vi "ConvertGoop3ToGoop4_UpdateGetAttributes.vi"(8 "error in (no error)":errorcluster, 10 "BaseClasses":path[](array[path]), 11 "ViRef":refnum<vi>) -> (0 "error out":errorcluster, 3 "ViRefOut":refnum<vi>)   [LabVIEW 2014]
uses:
  <resource>/Framework/Providers/Open_GDS/ClassProviders/Common/ScriptingFunctions/Scripting_FollowWireDownStreams_StopCriteria.ctl
panel:
  out "BundlerNames":cluster{"FullElemNms[]":cluster{string[]}[]}[](array[cluster])
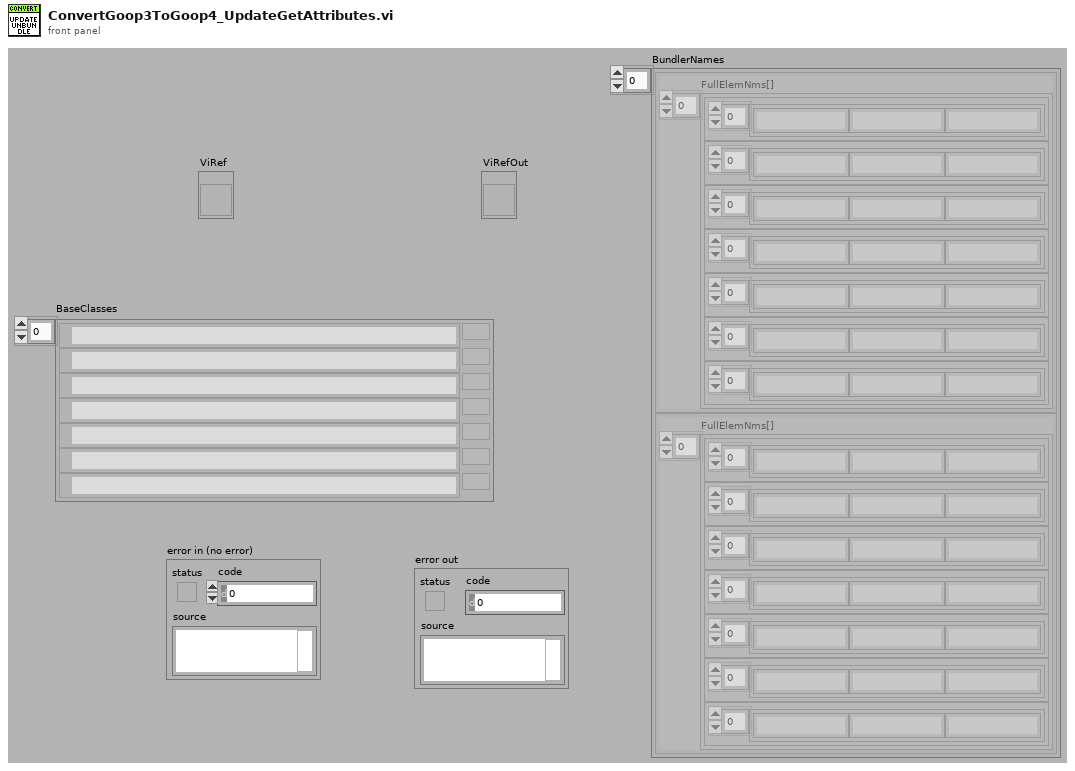
[diagram p1: front panel]
types:
  T1 = typedef "Scripting_FollowWireDownStreams_StopCriteria.ctl" = cluster{"ReachedANyOfTheseNodes":refnum<vi>[], "NodeType":string[], "VINames":string[], "AddTheseNodes":bool, "ALsoSerachOtherDrainNodes":bool}
  T2 = cluster{"Bundlers":refnum<vi>, "BundlersSourceTerms":refnum<vi>[], "BundlersClassBelongingsOut":i32[], "Bundler":refnum<vi>}[]
  T3 = cluster{"WhileLoop":refnum<vi>, refnum<vi>[], i32[], "WhileLoop":refnum<vi>}
  T4 = cluster{"WhileLoop":refnum<vi>, "BundlersSourceTerms":refnum<vi>[], "BundlersClassBelongingsOut":i32[], "WhileLoop":refnum<vi>}[]
  T5 = cluster{"WhileLoop":refnum<vi>, "BundlersSourceTerms":refnum<vi>[], "BundlersClassBelongingsOut":i32[], "WhileLoop":refnum<vi>}
  T6 = cluster{"Bundlers":refnum<vi>, "BundlersSourceTerms":refnum<vi>[], "BundlersClassBelongingsOut":i32[], "Bundler":refnum<vi>}
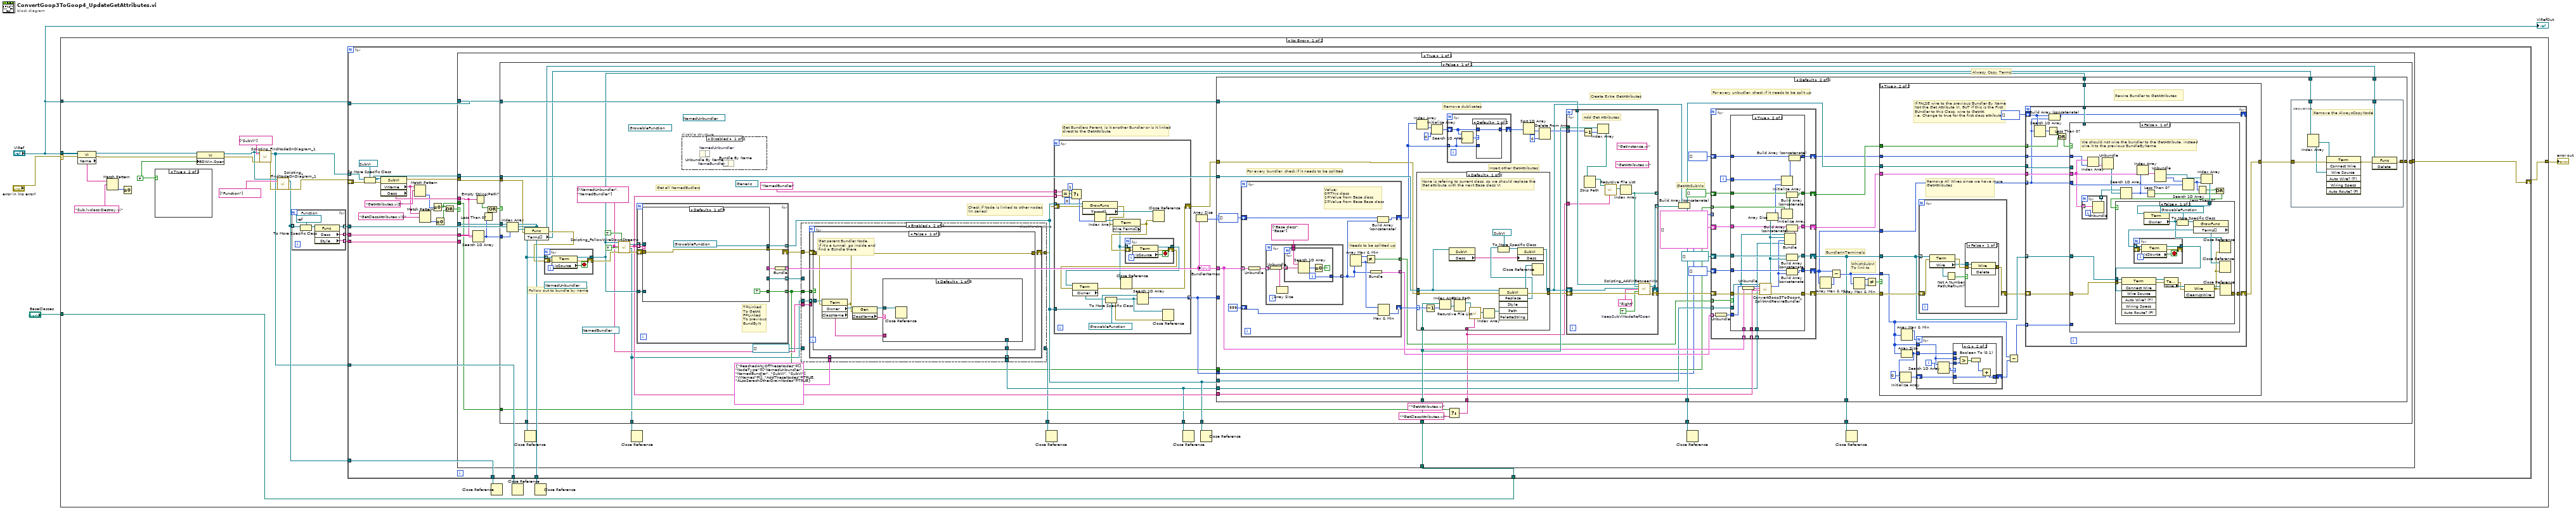
[diagram p0: block diagram]
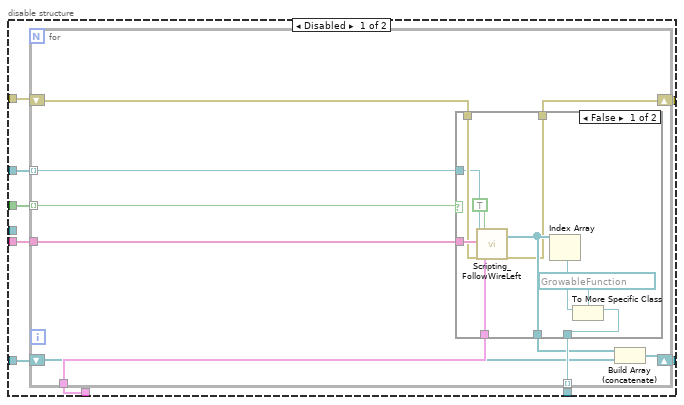
[diagram p4: hidden frame]
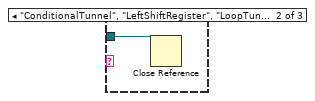
[diagram p6: hidden frame]
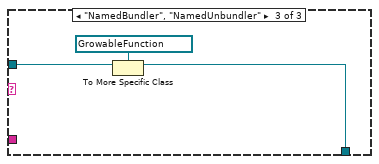
[diagram p7: hidden frame]
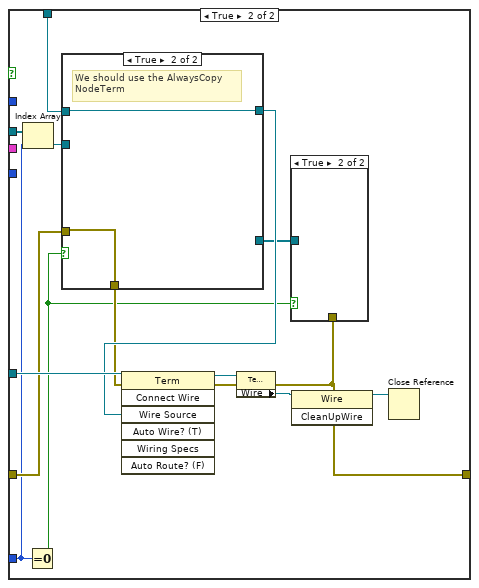
[diagram p13: hidden frame]
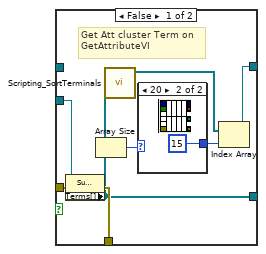
[diagram p14: hidden frame]
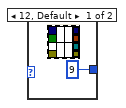
[diagram p15: hidden frame]
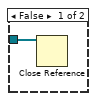
[diagram p16: hidden frame]
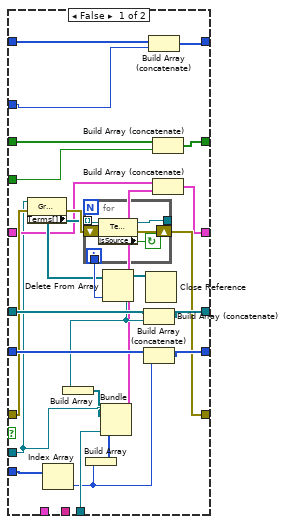
[diagram p18: hidden frame]
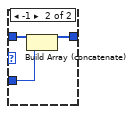
[diagram p19: hidden frame]
diagram:
  n1 = case shown="No Error" "error in (no error)" {
    selector: "error in (no error)" -> [w6 w587]
    tunnel: [w28 w587] -> w4
    tunnel: "ViRef" -> [w9 _]
    tunnel: "BaseClasses" -> [w15 _]
    tunnel: "ViRef" -> [w14 _]
    frame No Error {
      w5 = FALSE
      n2 = property class="VI"(reference=w9, error in=w6) -> (reference out=w8:refnum<vi>, error out=w7:errorcluster, "Name"=w12:string)
      n3 = Match Pattern(string=w12, regular expression="Sub.lvclass:Destroy.vi") -> (offset past match=w10:i32)  [unwired: 1 in, 3 out]
      n4 = Greater Or Equal To 0?(x=w10) -> ()  [unwired: 1 out]
      n5 = case shown="True" w5 {
        frame False {
        }
        frame True {
        }
      }
      n6 = property class="VI"(reference=w8, error in=w7, "BDWin.Open"=w5) -> (reference out=w26:refnum<vi>, error out=w27:errorcluster)
      n7 = call <resource>:"Scripting_FindNodeOnDiagram_1.vi"("ViRef(Ignored If Not Wired)"=w26, "NodeTypesToSearchFor"=string[] ["SubVI"], "error in (no error)"=w27) -> ("Nodes"=w13:refnum<vi>[], "error out"=w24:errorcluster)  [unwired: 15 in]
      n8 = call <resource>:"Scripting_FindNodeOnDiagram_1.vi"("ViRef(Ignored If Not Wired)"=w26, "NodeTypesToSearchFor"=string[] ["Function"], "error in (no error)"=w24) -> ("Nodes"=w19:refnum<vi>[], "error out"=w23:errorcluster)  [unwired: 15 in]
      n9 = for {
        tunnel: w19 -> [w33] mode=indexing
        tunnel: [w32] -> w22 mode=indexing
        tunnel: [w31] -> w21 mode=indexing
        tunnel: [w30] -> w16 mode=indexing
        w34 = refnum<vi> refnum  # Function
        n10 = To More Specific Class(target class=w34, reference=w33) -> (specific class reference=w35:refnum<vi>)  [unwired: 1 in, 1 out]
        n11 = property class="Func"(reference=w35) -> (reference out=w31:refnum<vi>, "Desc"=w32:string, "Style"=w30:string)  [unwired: 1 in, 1 out]
      }
      n12 = for {
        tunnel: w13 -> [w59] mode=indexing
        shift-right: [w46] -> w28
        shift-left: w23 -> [w57]
        tunnel: w22 -> [w50]
        tunnel: w21 -> [w49]
        tunnel: [w49] -> w20
        tunnel: w19 -> [w48]
        tunnel: [w48] -> w18
        tunnel: w13 -> [w47]
        tunnel: [w47] -> w17
        tunnel: w16 -> [w45]
        tunnel: w15 -> [w44]
        tunnel: w14 -> [w43]
        n13 = To More Specific Class(target class=refnum<vi> refnum ("WhileLoop"), reference=w59, error in=w57) -> (specific class reference=w56:refnum<vi>, error out=w55:errorcluster)
        n14 = property class="SubVI"(reference=w56, error in=w55) -> (reference out=w53:refnum<vi>, error out=w52:errorcluster, "VIName"=w36:string, "Desc"=w51:string)
        n15 = Match Pattern(string=w36, regular expression="GetAttributes.vi$") -> (offset past match=w39:i32)  [unwired: 1 in, 3 out]
        n16 = Match Pattern(string=w36, regular expression="GetClassAttributes.vi$") -> (offset past match=w41:i32)  [unwired: 1 in, 3 out]
        n17 = Greater Or Equal To 0?(x=w39) -> (x >= 0?=w37:bool)
        n18 = Greater Or Equal To 0?(x=w41) -> (x >= 0?=w40:bool)
        n19 = Or(x=w37, y=w40) -> (x .or. y?=w38:bool)
        n20 = case shown="True" w38 {
          tunnel: w53 -> [w79 _]
          tunnel: w52 -> [w78 w586]
          tunnel: [w77 w586] -> w46
          tunnel: w51 -> [w72 _]
          tunnel: w50 -> [w76 _]
          tunnel: w49 -> [w75 _]
          tunnel: w45 -> [_ _]
          tunnel: w44 -> [w74 _]
          tunnel: w43 -> [w73 _]
          tunnel: w37 -> [w63 _]
          frame True {
            n21 = Search 1D Array(1D array=w76, element=w72) -> (index of element=w70:i32)  [unwired: 1 in]
            n22 = Empty String/Path?(string/path=w72) -> (empty?=w71:bool)
            n23 = Less Than 0?(x=w70) -> (x < 0?=w69:bool)
            n24 = Compound Arithmetic op=OR(w71, w69) -> (w68:bool)
            n25 = case shown="False" w68 {
              tunnel: w79 -> [w114 _]
              tunnel: w78 -> [w96 w585]
              tunnel: [w109 w585] -> w77
              tunnel: w75 -> [w119 _]
              tunnel: w74 -> [w112 _]
              tunnel: w73 -> [w113 _]
              tunnel: w70 -> [w110 _]
              tunnel: [w107 _] -> w67
              tunnel: [w97 _] -> w66
              tunnel: [w106 _] -> w65
              tunnel: [w105 _] -> w64
              tunnel: w63 -> [w94 _]
              tunnel: [w90 _] -> w62
              tunnel: [w85 _] -> w61
              tunnel: [w84 _] -> w60
              frame False {
                (unwired) refnum<vi> refnum ("Owner")
                (unwired) refnum<vi> refnum ("WhileLoop")
                (unwired) refnum<vi> refnum ("WhileLoop")
                (unwired) refnum<vi> refnum ("WhileLoop")
                w88 = string[] ["NamedUnbundler", "NamedBundler"]
                (unwired) refnum<vi> refnum ("WhileLoop")
                # "Check if Node is linked to other nodes\n(In series)"
                # "Get Bundlers Parent, is it another Bundler or is it linked\ndirect to the GetAttribute"
                # "Alwasy Copy Terms"
                # "Get all NamedBudlers"
                # "Follow out to bundle by name"
                n26 = Index Array(array=w119, index=w110) -> (element=w118:refnum<vi>)
                n27 = property class="Func"(reference=w118, error in=w96) -> (reference out=w108:refnum<vi>, error out=w116:errorcluster, "Terms[]"=w107:refnum<vi>[])
                n28 = for {
                  tunnel: w107 -> [w533] mode=indexing
                  tunnel: [w532] -> w102
                  shift-right: [w529] -> w115
                  shift-left: w116 -> [w530]
                  stop <- w531 stop-if-true
                  n29 = property class="Term"(reference=w533, error in=w530) -> (reference out=w532:refnum<vi>, error out=w529:errorcluster, "IsSource"=w531:bool)
                }
                n30 = call <resource>:"Scripting_FollowWireDownStreams.vi"("Term Refnum"=w102, "NodeTypesToFind"=w88, "CreateParentTerminals(False)"=TRUE, "error in"=w115, "MainitainDataType"=TRUE ("MainitainDateType(True)")) -> ("Nodes"=w111:refnum<vi>[], "NodeTypes"=w101:string[], "ParentTerminal"=w84:refnum<vi>[], "error out"=w117:errorcluster)  [unwired: 11 in]
                n31 = for {
                  tunnel: w111 -> [w543] mode=indexing
                  shift-right: [w541] -> w89
                  shift-left: w117 -> [w542]
                  tunnel: [w539] -> w104 mode=indexing
                  tunnel: [w537] -> w97 mode=indexing
                  tunnel: w101 -> [w538] mode=indexing
                  tunnel: w102 -> [w536]
                  tunnel: [w535] -> w83 mode=indexing
                  tunnel: [w534] -> w82 mode=indexing
                  # "T=Linked\nTo GetAt\nF=Linked\nTo previous\nBundByN"
                  n32 = case shown="Default" w538 {
                    tunnel: w543 -> [_ w565 w584]
                    tunnel: w542 -> [w546 w561 w581]
                    tunnel: [w546 w560 w580] -> w541
                    tunnel: [_ w559 w579] -> w540
                    tunnel: [refnum<vi> refnum ("WhileLoop") w556 w576] -> w537
                    tunnel: w536 -> [_ w554 w574]
                    tunnel: [TRUE w552 w572] -> w535
                    tunnel: [_ w547 w568] -> w534
                    frame Default {
                    }
                    frame "NamedUnbundler" {
                      (unwired) refnum<vi> refnum ("WhileLoop")
                      n33 = To More Specific Class(target class=refnum<vi> refnum ("WhileLoop"), reference=w565, error in=w561) -> (specific class reference=w563:refnum<vi>, error out=w562:errorcluster)
                      n34 = property class="NmdUnbndl"(reference=w563, error in=w562) -> (reference out=w558:refnum<vi>, error out=w560:errorcluster, "FullElemNms[]"=w559:cluster{string[]}[], "Terms[]"=w551:refnum<vi>[])
                      n35 = Delete From Array(array=w551, index=0) -> (deleted portion=w548:refnum<vi>, array with subset deleted=w550:refnum<vi>[])  [unwired: 1 in]
                      n36 = property class="Term"(reference=w548) -> (reference out=w547:refnum<vi>, "Wire.Terms[]"=w555:refnum<vi>[])  [unwired: 1 in, 1 out]
                      n37 = To More Generic Class(target class=refnum<vi> refnum ("WhileLoop"), reference=w558) -> (generic class reference=w556:refnum<vi>)
                      n38 = Search 1D Array(1D array=w555, element=w554) -> (index of element=w553:i32)  [unwired: 1 in]
                      n39 = Close Reference(reference=w555) -> ()  [unwired: 1 in, 1 out]
                      n40 = Greater Or Equal To 0?(x=w553) -> (x >= 0?=w552:bool)
                      n41 = Close Reference(reference=w550) -> ()  [unwired: 1 in, 1 out]
                    }
                    frame "NamedBundler" {
                      n42 = To More Specific Class(target class=refnum<vi> refnum ("WhileLoop"), reference=w584, error in=w581) -> (specific class reference=w583:refnum<vi>, error out=w582:errorcluster)
                      n43 = property class="NmdBndl"(reference=w583, error in=w582) -> (reference out=w577:refnum<vi>, error out=w580:errorcluster, "FullElemNms[]"=w579:cluster{string[]}[], "Terms[]"=w566:refnum<vi>[])
                      n44 = Delete From Array(array=w566, index=1) -> (deleted portion=w569:refnum<vi>, array with subset deleted=w567:refnum<vi>[])  [unwired: 1 in]
                      n45 = property class="Term"(reference=w569) -> (reference out=w568:refnum<vi>, "Wire.Terms[]"=w571:refnum<vi>[])  [unwired: 1 in, 1 out]
                      n46 = To More Generic Class(target class=refnum<vi> refnum ("WhileLoop"), reference=w577) -> (generic class reference=w576:refnum<vi>)
                      n47 = Search 1D Array(1D array=w571, element=w574) -> (index of element=w573:i32)  [unwired: 1 in]
                      n48 = Greater Or Equal To 0?(x=w573) -> (x >= 0?=w572:bool)
                      n49 = Close Reference(reference=w571) -> ()  [unwired: 1 in, 1 out]
                      n50 = Close Reference(reference=w567) -> ()  [unwired: 1 in, 1 out]
                    }
                  }
                  n51 = Bundle("FullElemNms[]"=w540) -> (w539:cluster{"FullElemNms[]":cluster{string[]}[]})  [unwired: 1 in]
                }
                "BundlerNames" <- w104
                n52 = disable-structure shown="Disabled" {
                  frame Disabled {
                    n53 = Unbundle By Name "NamedUnbundler"() -> ()  [unwired: 1 in, 1 out]
                    n54 = Bundle By Name "NameBundler"() -> ()  [unwired: 2 in, 1 out]
                  }
                  frame Enabled {
                  }
                }
                n55 = disable-structure shown="Enabled" {
                  disable-tunnel: [w127 w155] -> w90
                  disable-tunnel: w89 -> [w126 w154]
                  disable-tunnel: w88 -> [w125 w153]
                  disable-tunnel: T1 {"ReachedANyOfTheseNodes"=[], "NodeType"=["NamedUnbundler", "NamedBundler", "SubVI", "SubVI"], "VINames"=[], "AddTheseNodes"=TRUE, "ALsoSerachOtherDrainNodes"=TRUE} ("StopCriteria") -> [w124 w152]
                  disable-tunnel: refnum<vi>[] [] -> [w123 _]
                  disable-tunnel: [w122 _] -> w85
                  disable-tunnel: w84 -> [_ w151]
                  disable-tunnel: w83 -> [w121 w149]
                  disable-tunnel: w82 -> [w120 _]
                  disable-tunnel: [_ w150] -> w81
                  frame Disabled {
                    n56 = for {
                      tunnel: [w137] -> w127 mode=indexing
                      shift-right: [w130] -> _
                      shift-left: w126 -> [w131]
                      tunnel: w125 -> [w136]
                      tunnel: w124 -> [w135]
                      shift-right: [w132] -> w122
                      shift-left: w123 -> [w133]
                      tunnel: w121 -> [w129] mode=indexing
                      tunnel: w120 -> [w128] mode=indexing
                      n57 = case shown="False" w129 {
                        tunnel: [w147 _] -> w137
                        tunnel: w136 -> [w146 _]
                        tunnel: w135 -> [w145 _]
                        tunnel: [w144 _] -> w134
                        tunnel: w131 -> [w141 w148]
                        tunnel: [w140 w148] -> w130
                        tunnel: w128 -> [w138 _]
                        frame False {
                          n58 = call <resource>:"Scripting_FollowWireLeft.vi"("Term Refnum"=w138, "NodeTypesToFind"=w146, "error in"=w141, "MainitainDataType"=TRUE, "StopCriteria"=w145) -> ("Nodes"=w144:refnum<vi>[], "error out"=w140:errorcluster)  [unwired: 11 in, 2 out]
                          n59 = Index Array(array=w144) -> (element=w142:refnum<vi>)  [unwired: 1 in]
                          n60 = To More Specific Class(target class=refnum<vi> refnum ("WhileLoop"), reference=w142) -> (specific class reference=w147:refnum<vi>)  [unwired: 1 in, 1 out]
                        }
                        frame True {
                        }
                      }
                      n61 = Build Array (concatenate)(w134, w133) -> (w132:refnum<vi>[])
                    }
                  }
                  frame Enabled {
                    n62 = for {
                      tunnel: w151 -> [w160] mode=indexing
                      tunnel: [w159] -> w155 mode=indexing
                      shift-right: [w158] -> w150
                      shift-left: w154 -> [w157]
                      tunnel: w153 -> [_]
                      tunnel: w152 -> [_]
                      tunnel: w149 -> [w156] mode=indexing
                      n63 = case shown="False" w156 {
                        tunnel: w160 -> [w168 _]
                        tunnel: [w166 _] -> w159
                        tunnel: [w161 w174] -> w158
                        tunnel: w157 -> [w167 w174]
                        frame False {
                          # "Get parent Bundler Node,\nif it's a tunnel, go inside and\nfind a BUndle there"
                          n64 = property class="Term"(reference=w168, error in=w167) -> (error out=w161:errorcluster, "Owner"=w163:refnum<vi>, "ClassName"=w165:string)  [unwired: 1 out]
                          n65 = property class="Gen"(reference=w163, error in=w161) -> (reference out=w162:refnum<vi>, "ClassName"=w164:string)  [unwired: 1 out]
                          n66 = case shown="Default" w164 {
                            tunnel: w162 -> [w169 w170 w172]
                            tunnel: [_ _ w171] -> w166
                            tunnel: w165 -> [_ _ _]
                            frame Default {
                              n67 = Close Reference(reference=w169) -> ()  [unwired: 1 in, 1 out]
                            }
                            frame "ConditionalTunnel", "LeftShiftRegister", "LoopTunnel", "RightShiftRegister", "SelectorTunnel", "Tunnel" {
                              n68 = Close Reference(reference=w170) -> ()  [unwired: 1 in, 1 out]
                            }
                            frame "NamedBundler", "NamedUnbundler" {
                              n69 = To More Specific Class(target class=refnum<vi> refnum ("WhileLoop"), reference=w172) -> (specific class reference=w171:refnum<vi>)  [unwired: 1 in, 1 out]
                            }
                          }
                        }
                        frame True {
                        }
                      }
                    }
                  }
                }
                n70 = for {
                  tunnel: w97 -> [w195] mode=indexing
                  tunnel: w101 -> [w197] mode=indexing
                  tunnel: "NamedBundler" ("regular expression") -> [w196]
                  tunnel: w97 -> [w187]
                  tunnel: [w184] -> w99 mode=indexing
                  shift-right: [w178] -> w80
                  shift-left: w81 -> [w183]
                  n71 = Equal?(x=w196, y=w197) -> (x = y?=w194:bool)
                  n72 = Select(t=1 ("index"), s=w194, f=0 ("index")) -> (s? t:f=w193:i32)
                  n73 = property class="GrowFunc"(reference=w195, error in=w183) -> (error out=w180:errorcluster, "Terms[]"=w181:refnum<vi>[])  [unwired: 1 out]
                  n74 = Index Array(array=w181, index=w193) -> (element=w190:refnum<vi>)
                  n75 = property class="Term"(reference=w190, error in=w180) -> (error out=w182:errorcluster, "Wire.Terms[]"=w177:refnum<vi>[])  [unwired: 1 out]
                  n76 = for {
                    tunnel: w177 -> [w202] mode=indexing
                    tunnel: [w201] -> w189
                    shift-right: [w198] -> w188
                    shift-left: w182 -> [w199]
                    stop <- w200 stop-if-true
                    n77 = property class="Term"(reference=w202, error in=w199) -> (reference out=w201:refnum<vi>, error out=w198:errorcluster, "IsSource"=w200:bool)
                  }
                  n78 = property class="Term"(reference=w189, error in=w188) -> (error out=w179:errorcluster, "Owner"=w186:refnum<vi>)  [unwired: 1 out]
                  n79 = To More Specific Class(target class=refnum<vi> refnum ("WhileLoop"), reference=w186) -> (specific class reference=w175:refnum<vi>, error out=w176:errorcluster)  [unwired: 1 in]
                  n80 = Close Reference(reference=w177, error in (no error)=w179) -> (error out=w178:errorcluster)
                  n81 = Search 1D Array(1D array=w187, element=w175) -> (index of element=w184:i32)  [unwired: 1 in]
                  n82 = Close Reference(reference=w181, error in (no error)=w182) -> ()  [unwired: 1 out]
                  n83 = Close Reference(reference=w175, error in (no error)=w176) -> ()  [unwired: 1 out]
                }
                n84 = Array Size(array=w104) -> (size(s)=w103:i32)
                n85 = Select(t="*GetAttributes.vi" ("pattern"), s=w94, f="*GetClassAttributes.vi" ("pattern")) -> (s? t:f=w92:string)
                n86 = case shown="Default" w103 {
                  tunnel: w114 -> [_ w251]
                  tunnel: w113 -> [_ w241]
                  tunnel: w112 -> [_ w240]
                  tunnel: w104 -> [_ w237]
                  tunnel: w80 -> [w203 w226]
                  tunnel: [w203 w224] -> w109
                  tunnel: w108 -> [_ w223]
                  tunnel: w102 -> [_ w222]
                  tunnel: w107 -> [_ w221]
                  tunnel: w97 -> [_ w220]
                  tunnel: [_ w219] -> w106
                  tunnel: [_ w218] -> w105
                  tunnel: w101 -> [_ w217]
                  tunnel: w83 -> [_ w214]
                  tunnel: w99 -> [_ _]
                  tunnel: w99 -> [_ w211]
                  tunnel: w90 -> [_ w205]
                  tunnel: w92 -> [_ w204]
                  frame 0 {
                  }
                  frame Default {
                    # "WhichSubVI\nTo link to"
                    # "BundlerInTerminals"
                    # "GetAttrSubVIs"
                    # "For every bundler, check if it needs to be splitted"
                    # "For every unbudler, check if it needs to be split up"
                    # "Create Extra GetAttributes"
                    # "Remove dublicates"
                    # "Insert other GetAttributes"
                    n87 = for {
                      tunnel: w237 -> [w519] mode=indexing
                      tunnel: [w515] -> w239 mode=indexing
                      tunnel: [w514] -> w238 mode=indexing
                      shift-right: [w511] -> w252
                      shift-left: 999 -> [w512]
                      shift-right: [w510] -> w246
                      shift-left: i32[] [] -> [w509]
                      # "Needs to be splitted up"
                      # "Value:\n0=This class\n1=Value from Base class\n2=Value from Base Base class"
                      n88 = Unbundle(w519) -> ("FullElemNms[]"=w518:cluster{string[]}[])
                      n89 = for {
                        tunnel: w518 -> [w523] mode=indexing
                        tunnel: string[] ["Base class", "Base"] ("1D array") -> [w522]
                        tunnel: [w520] -> w508 mode=indexing
                        n90 = Unbundle(w523) -> (w521:string[])
                        n91 = Array Size(array=w521) -> ()  [unwired: 1 out]
                        n92 = for {
                          tunnel: w521 -> [w528] mode=indexing
                          tunnel: w522 -> [w527]
                          tunnel: [w524] -> w520
                          i -> [w524]
                          stop <- w525 continue-if-true
                          n93 = Search 1D Array(1D array=w527, element=w528) -> (index of element=w526:i32)  [unwired: 1 in]
                          n94 = Greater Or Equal To 0?(x=w526) -> (x >= 0?=w525:bool)
                        }
                      }
                      n95 = Array Max & Min(array=w508) -> (max value=w516:i32, min value=w513:i32)  [unwired: 2 out]
                      n96 = Not Equal?(x=w516, y=w513) -> (x != y?=w515:bool)
                      n97 = Bundle(w508) -> (w514:cluster{i32[]})  [unwired: 1 in]
                      n98 = Build Array (concatenate)(w509, w508) -> (w510:i32[])
                      n99 = Max & Min(x=w513, y=w512) -> (min(x,y)=w511:i32)  [unwired: 1 out]
                    }
                    n100 = case shown="Default" w252 {
                      selector: w252 -> [w504 _]
                      tunnel: w240 -> [w503 _]
                      tunnel: w251 -> [w495 w506]
                      tunnel: w226 -> [w502 w507]
                      tunnel: [w501 w507] -> w216
                      tunnel: [w489 w506] -> w233
                      tunnel: w204 -> [w496 _]
                      frame Default {
                        # "None is refering to current class, so we should replace the\nGet attribute with the next Base class VI"
                        n101 = Decrement(x=w504) -> (x-1=w505:i32)
                        n102 = Index Array(array=w503, index=w505) -> (element=w500:path)
                        n103 = property class="SubVI"(reference=w495) -> ("Desc"=w490:string)  [unwired: 1 in, 2 out]
                        n104 = Strip Path(path=w500) -> (stripped path=w499:path)  [unwired: 1 out]
                        n105 = call <vilib>:"Recursive File List.vi"("pattern"=w496, "Folder Path"=w499) -> ("All Files in Dir"=w498:path[])  [unwired: 5 in, 4 out]
                        n106 = Index Array(array=w498) -> (element=w497:path)  [unwired: 1 in]
                        n107 = invoke class="SubVI" method="Replace"(reference=w495, error in=w502, "Path"=w497) -> (reference out=w494:refnum<vi>, error out=w501:errorcluster, "Replace"=w492:refnum<vi>)  [unwired: 3 in, 3 out]
                        n108 = To More Specific Class(target class=refnum<vi> refnum ("WhileLoop"), reference=w492) -> (specific class reference=w491:refnum<vi>)  [unwired: 1 in, 1 out]
                        n109 = property class="SubVI"(reference=w491, "Desc"=w490) -> (reference out=w489:refnum<vi>)  [unwired: 1 in, 1 out]
                        n110 = Close Reference(reference=w494) -> ()  [unwired: 1 in, 1 out]
                      }
                      frame 0 {
                        # "Some if refering to\nthe Current sub class\nSo keep the Current GetAttribute."
                      }
                    }
                    n111 = Index Array(array=w246) -> (element=w247:i32)  [unwired: 1 in]
                    n112 = Initialize Array(w247, 0 ("Dimension Size")) -> (w248:i32[])
                    n113 = for {
                      tunnel: w246 -> [w483] mode=indexing
                      shift-right: [w482] -> w245
                      shift-left: w248 -> [w481]
                      n114 = Search 1D Array(1D array=w481, element=w483) -> (index of element=w484:i32)  [unwired: 1 in]
                      n115 = case shown="Default" w484 {
                        tunnel: w483 -> [_ w488]
                        tunnel: [w485 w486] -> w482
                        tunnel: w481 -> [w485 w487]
                        frame Default {
                        }
                        frame -1 {
                          n116 = Build Array (concatenate)(w487, w488) -> (w486:i32[])
                        }
                      }
                    }
                    n117 = Sort 1D Array(array=w245) -> (sorted array=w244:i32[])
                    n118 = Delete From Array(array=w244, index=0) -> (array with subset deleted=w242:i32[])  [unwired: 1 in, 1 out]
                    n119 = for {
                      tunnel: w242 -> [w476] mode=indexing
                      shift-right: [w479] -> w215
                      shift-left: w216 -> [w480]
                      tunnel: w241 -> [w478]
                      tunnel: w240 -> [w475]
                      shift-right: [w467] -> _
                      shift-left: w233 -> [w471]
                      tunnel: [w468] -> _ mode=indexing
                      tunnel: [w467] -> w234 mode=indexing
                      tunnel: w204 -> [w466]
                      w470 = TRUE  # KeepSubVINodeRefOpen
                      (unwired) "GetAttributes.vi" ("regular expression")
                      (unwired) "GetInstance.vi" ("regular expression")
                      # "Add Get Attributes"
                      n120 = Decrement(x=w476) -> (x-1=w477:i32)
                      n121 = Index Array(array=w475, index=w477) -> (element=w469:path)
                      n122 = Strip Path(path=w469) -> (stripped path=w474:path)  [unwired: 1 out]
                      n123 = call <vilib>:"Recursive File List.vi"("pattern"=w466, "Folder Path"=w474) -> ("All Files in Dir"=w473:path[])  [unwired: 5 in, 4 out]
                      n124 = Index Array(array=w473) -> (element=w468:path)  [unwired: 1 in]
                      n125 = call <resource>:"Scripting_AddVIBetweenVIs.vi"("ViToModify"=w478, "VIToAdd"=w468, "VIOne(Path,Name or NamePattern)"=w471, "VITwo(Path,Name or NamePattern), If Left/Right-string, it will be placed to the right or left of VIOne"="Right" ("pattern"), "KeepSubVINodeRefOpen(False)"=w470, "error in (no error)"=w480) -> ("SubVI Refnum"=w467:refnum<vi>, "error out"=w479:errorcluster)  [unwired: 12 in]
                    }
                    n126 = Build Array (concatenate)(w233, w234) -> (w219:refnum<vi>[])
                    n127 = for {
                      shift-right: [w405] -> w231
                      shift-left: w215 -> [w406]
                      tunnel: w220 -> [w404] mode=indexing
                      tunnel: w239 -> [w407] mode=indexing
                      tunnel: w238 -> [w398] mode=indexing
                      tunnel: w237 -> [w403] mode=indexing
                      shift-right: [w401] -> w218
                      shift-left: refnum<vi>[] [] -> [w402]
                      shift-right: [w400] -> w208
                      shift-left: i32[] [] -> [w399]
                      tunnel: w217 -> [w396] mode=indexing
                      tunnel: w214 -> [w395] mode=indexing
                      shift-right: [w394] -> w212
                      shift-left: bool[] [] -> [w393]
                      tunnel: w211 -> [_] mode=indexing
                      shift-right: [w391] -> w209
                      shift-left: T2 [] -> [w392]
                      tunnel: w205 -> [w390] mode=indexing
                      shift-right: [w387] -> w206
                      shift-left: i32[] [] -> [w388]
                      i -> [w389]
                      n128 = Unbundle(w398) -> (w397:i32[])
                      n129 = case shown="True" w407 {
                        tunnel: w406 -> [w427 w465]
                        tunnel: [w426 w464] -> w405
                        tunnel: w404 -> [w414 w445]
                        tunnel: w403 -> [_ w463]
                        tunnel: w402 -> [w433 w461]
                        tunnel: [w432 w460] -> w401
                        tunnel: w399 -> [w429 w458]
                        tunnel: [w430 w459] -> w400
                        tunnel: w397 -> [w431 w457]
                        tunnel: w396 -> [_ w456]
                        tunnel: w395 -> [w420 w455]
                        tunnel: [w421 w454] -> w394
                        tunnel: w393 -> [w422 w453]
                        tunnel: [w415 w448] -> w391
                        tunnel: w392 -> [w416 w449]
                        tunnel: w390 -> [w413 w446]
                        tunnel: w389 -> [w417 w443]
                        tunnel: w388 -> [w419 w441]
                        tunnel: [w418 w440] -> w387
                        frame False {
                          n130 = property class="GrowFunc"(reference=w414, error in=w427) -> (error out=w428:errorcluster, "Terms[]"=w424:refnum<vi>[])  [unwired: 1 out]
                          n131 = Index Array(array=w431) -> (element=w412:i32)  [unwired: 1 in]
                          n132 = for {
                            tunnel: w424 -> [w439] mode=indexing
                            tunnel: [w438] -> _
                            shift-right: [w436] -> w426
                            shift-left: w428 -> [w437]
                            tunnel: [w434] -> w425
                            i -> [w434]
                            stop <- w435 continue-if-true
                            n133 = property class="Term"(reference=w439, error in=w437) -> (reference out=w438:refnum<vi>, error out=w436:errorcluster, "IsSource"=w435:bool)
                          }
                          n134 = Build Array(w412) -> (w411:i32[])
                          n135 = Delete From Array(array=w424, index=w425) -> (deleted portion=w410:refnum<vi>, array with subset deleted=w423:refnum<vi>[])  [unwired: 1 in]
                          n136 = Build Array(w410) -> (w409:refnum<vi>[])
                          n137 = Bundle("WhileLoop"=w414, w409, w411, "WhileLoop"=w413) -> (w408:T3)  [unwired: 1 in]
                          n138 = Build Array (concatenate)(w433, w410) -> (w432:refnum<vi>[])
                          n139 = Build Array (concatenate)(w429, w412) -> (w430:i32[])
                          n140 = Close Reference(reference=w423) -> ()  [unwired: 1 in, 1 out]
                          n141 = Build Array (concatenate)(w419, w417) -> (w418:i32[])
                          n142 = Build Array (concatenate)(w422, w420) -> (w421:bool[])
                          n143 = Build Array (concatenate)(w416, w408) -> (w415:T4)
                        }
                        frame True {
                          n144 = Unbundle(w463) -> ("FullElemNms[]"=w462:cluster{string[]}[])
                          n145 = call <resource>:"ConvertGoop3ToGoop4_SplitAndRewireBundler.vi"("UnBundlerOrBundler"=w445, "ClassBelongings"=w457, "FullElemNms[]"=w462, "TypeString"=w456, "error in (no error)"=w465) -> ("BundlersSourceTerms"=w451:refnum<vi>[], "BundlersClassBelongingsOut"=w450:i32[], "error out"=w464:errorcluster)  [unwired: 12 in]
                          n146 = Array Size(array=w451) -> (size(s)=w444:i32)
                          n147 = Initialize Array(w443, w444) -> (w442:i32[])
                          n148 = Initialize Array(w455, w444) -> (w452:bool[])
                          n149 = Bundle("WhileLoop"=w445, "BundlersSourceTerms"=w451, "BundlersClassBelongingsOut"=w450, "WhileLoop"=w446) -> (w447:T5)  [unwired: 1 in]
                          n150 = Build Array (concatenate)(w453, w452) -> (w454:bool[])
                          n151 = Build Array (concatenate)(w449, w447) -> (w448:T4)
                          n152 = Build Array (concatenate)(w461, w451) -> (w460:refnum<vi>[])
                          n153 = Build Array (concatenate)(w458, w450) -> (w459:i32[])
                          n154 = Build Array (concatenate)(w441, w442) -> (w440:i32[])
                        }
                      }
                    }
                    n155 = Array Max & Min(array=w208) -> (min value=w232:i32)  [unwired: 3 out]
                    n156 = Subtract(x=w208, y=w232) -> (x-y=w228:i32[])
                    n157 = Array Max & Min(array=w228) -> (max value=w230:i32, min value=w229:i32)  [unwired: 2 out]
                    n158 = Not Equal?(x=w230, y=w229) -> (x != y?=w227:bool)
                    n159 = case shown="True" w227 {
                      tunnel: w219 -> [_ w277]
                      tunnel: w218 -> [_ w278]
                      tunnel: w231 -> [w261 w279]
                      tunnel: [w261 w274] -> w225
                      tunnel: w228 -> [_ w262]
                      tunnel: w222 -> [_ w276]
                      tunnel: w212 -> [_ w273]
                      tunnel: w209 -> [_ w272]
                      tunnel: w208 -> [_ w271]
                      tunnel: w206 -> [_ w270]
                      frame False {
                        # "Only One GetAttribute"
                      }
                      frame True {
                        # "If FALSE wire to the previous Bundler By Name\nNot the Get Attribute VI, BUT if this is the First\nBUndler to this Class, wire to GetAtt.\ni.e. Change to true for the first class attribute"
                        # "Rewire Bundler to GetAttributes"
                        # "Remove All Wires since we have more GetAttributes"
                        n160 = Array Max & Min(array=w262) -> (max value=w264:i32)  [unwired: 3 out]
                        n161 = Array Size(array=w262) -> (size(s)=w265:i32)
                        n162 = Initialize Array(0, w265) -> (w266:i32[])
                        n163 = for {
                          N: w264 -> [_]
                          shift-right: [w280] -> w268
                          shift-left: w266 -> [w281]
                          tunnel: w265 -> [w283]
                          tunnel: w262 -> [w282]
                          i -> [w284]
                          n164 = Search 1D Array(1D array=w282, element=w284) -> (index of element=w285:i32)  [unwired: 1 in]
                          n165 = case shown="-1" w285 {
                            tunnel: w282 -> [_ w290]
                            tunnel: w284 -> [_ w292]
                            tunnel: w283 -> [_ _]
                            tunnel: w281 -> [w286 w288]
                            tunnel: [w286 w287] -> w280
                            frame 0, Default {
                            }
                            frame -1 {
                              n166 = Greater?(x=w290, y=w292) -> (0:w291:bool[])
                              n167 = Boolean To (0,1)(Boolean=w291) -> (0, 1=w289:i16[])
                              n168 = Add(x=w289, y=w288) -> (x+y=w287:i32[])
                            }
                          }
                        }
                        n169 = for {
                          tunnel: w278 -> [w382] mode=indexing
                          shift-right: [w379] -> w275
                          shift-left: w279 -> [w381]
                          n170 = property class="Term"(reference=w382, error in=w381) -> (error out=w380:errorcluster, "Wire"=w378:refnum<vi>)  [unwired: 1 out]
                          n171 = Not A Number/Path/Refnum?(number/path/refnum=w378) -> (NaN/Path/Refnum?=w377:bool)
                          n172 = case shown="False" w377 {
                            tunnel: w380 -> [w385 w386]
                            tunnel: [w384 w386] -> w379
                            tunnel: w378 -> [w383 _]
                            frame False {
                              n173 = invoke class="Wire" method="Delete"(reference=w383, error in=w385) -> (error out=w384:errorcluster)  [unwired: 1 in, 2 out]
                            }
                            frame True {
                            }
                          }
                        }
                        n174 = Subtract(x=w262, y=w268) -> (x-y=w263:i32[])
                        n175 = for {
                          tunnel: w278 -> [w303] mode=indexing
                          shift-right: [w307] -> w274
                          shift-left: w275 -> [w302]
                          tunnel: w277 -> [w306]
                          tunnel: w263 -> [w305] mode=indexing
                          tunnel: w276 -> [w304]
                          tunnel: w273 -> [w299] mode=indexing
                          tunnel: w272 -> [w301]
                          tunnel: w271 -> [w293] mode=indexing
                          tunnel: w270 -> [w300] mode=indexing
                          shift-right: [w294] -> _
                          shift-left: i32[] [] -> [w295]
                          n176 = Search 1D Array(1D array=w295, element=w293) -> (index of element=w297:i32)  [unwired: 1 in]
                          n177 = Less Than 0?(x=w297) -> (x < 0?=w296:bool)
                          n178 = Build Array (concatenate)(w295, w293) -> (w294:i32[])
                          n179 = Or(x=w296, y=w299) -> (x .or. y?=w298:bool)
                          n180 = case shown="False" w298 {
                            tunnel: [w325 w351] -> w307
                            tunnel: w306 -> [_ w363]
                            tunnel: w305 -> [_ w350]
                            tunnel: w304 -> [_ w361]
                            tunnel: w303 -> [w319 w360]
                            tunnel: w302 -> [w324 w358]
                            tunnel: w301 -> [w318 _]
                            tunnel: w293 -> [w322 _]
                            tunnel: w300 -> [w317 _]
                            frame False {
                              # "We should not wire the bundler to the GetAttribute, instead\nwire it to the previous BundleByName"
                              n181 = for {
                                tunnel: w318 -> [w348] mode=indexing
                                tunnel: [w347] -> w315 mode=indexing
                                n182 = Unbundle(w348) -> ("Bundlers"=w347:refnum<vi>)  [unwired: 3 out]
                              }
                              n183 = Index Array(array=w318, index=w317) -> (element=w316:T6)
                              n184 = Unbundle(w316) -> ("Bundler"=w314:refnum<vi>)  [unwired: 3 out]
                              n185 = Search 1D Array(1D array=w315, element=w314) -> (index of element=w312:i32)  [unwired: 1 in]
                              n186 = Index Array(array=w318, index=w312) -> (element=w323:T6)
                              n187 = Less Than 0?(x=w312) -> (x < 0?=w309:bool)
                              n188 = Unbundle(w323) -> ("BundlersSourceTerms"=w321:refnum<vi>[], "BundlersClassBelongingsOut"=w320:i32[])  [unwired: 2 out]
                              n189 = Search 1D Array(1D array=w320, element=w322) -> (index of element=w311:i32)  [unwired: 1 in]
                              n190 = Less Than 0?(x=w311) -> (x < 0?=w310:bool)
                              n191 = Index Array(array=w321, index=w311) -> (element=w313:refnum<vi>)
                              n192 = Or(x=w310, y=w309) -> (x .or. y?=w308:bool)
                              n193 = case shown="False" w308 {
                                tunnel: [w335 w346] -> w325
                                tunnel: w324 -> [w334 w346]
                                tunnel: w319 -> [w333 _]
                                tunnel: w313 -> [w331 _]
                                frame False {
                                n194 = property class="Term"(reference=w331) -> ("Owner"=w326:refnum<vi>)  [unwired: 1 in, 2 out]
                                n195 = To More Specific Class(target class=refnum<vi> refnum ("WhileLoop"), reference=w326) -> (specific class reference=w330:refnum<vi>)  [unwired: 1 in, 1 out]
                                n196 = property class="GrowFunc"(reference=w330) -> ("Terms[]"=w328:refnum<vi>[])  [unwired: 1 in, 2 out]
                                n197 = for {
                                tunnel: w328 -> [w345] mode=indexing
                                tunnel: [w344] -> w329
                                shift-right: [w341] -> _
                                shift-left: _ -> [w342]
                                stop <- w343 stop-if-true
                                n198 = property class="Term"(reference=w345, error in=w342) -> (reference out=w344:refnum<vi>, error out=w341:errorcluster, "IsSource"=w343:bool)
                                }
                                n199 = invoke class="Term" method="Connect Wire"(reference=w333, error in=w334, "Wire Source"=w329) -> (reference out=w340:refnum<vi>, error out=w339:errorcluster)  [unwired: 4 in, 5 out]
                                n200 = property class="Term"(reference=w340, error in=w339) -> (error out=w336:errorcluster, "Wire"=w338:refnum<vi>)  [unwired: 1 out]
                                n201 = invoke class="Wire" method="CleanUpWire"(reference=w338, error in=w336) -> (reference out=w337:refnum<vi>, error out=w327:errorcluster)  [unwired: 1 in, 1 out]
                                n202 = Close Reference(reference=w328, error in (no error)=w327) -> ()  [unwired: 1 out]
                                n203 = Close Reference(reference=w326, error in (no error)=w327) -> ()  [unwired: 1 out]
                                n204 = Close Reference(reference=w337, error in (no error)=w327) -> (error out=w335:errorcluster)
                                }
                                frame True {
                                }
                              }
                            }
                            frame True {
                              n205 = Index Array(array=w363, index=w350) -> (element=w362:refnum<vi>)
                              n206 = Equal To 0?(x=w350) -> (x = 0?=w349:bool)
                              n207 = case shown="True" w349 {
                                tunnel: w362 -> [w367 _]
                                tunnel: w361 -> [_ w375]
                                tunnel: [w368 w375] -> w359
                                tunnel: w358 -> [w366 w374]
                                tunnel: [w365 w374] -> w357
                                tunnel: [w364 _] -> w356
                                frame False {
                                # "Get Att cluster Term on\nGetAttributeVI"
                                n208 = property class="SubVI"(reference=w367, error in=w366) -> (error out=w365:errorcluster, "Terms[]"=w364:refnum<vi>[])  [unwired: 1 out]
                                n209 = Array Size(array=w364) -> (size(s)=w371:i32)
                                n210 = call <resource>:"Scripting_SortTerminals.vi"("Terminals[]"=w364) -> ("TerminalsOut[]"=w369:refnum<vi>[])  [unwired: 8 in, 2 out]
                                n211 = case shown="20" w371 {
                                tunnel: [9 ("index") 15 ("index")] -> w370
                                frame 12, Default {
                                }
                                frame 20 {
                                }
                                }
                                n212 = Index Array(array=w369, index=w370) -> (element=w368:refnum<vi>)
                                }
                                frame True {
                                # "We should use the AlwaysCopy\nNodeTerm"
                                }
                              }
                              n213 = invoke class="Term" method="Connect Wire"(reference=w360, error in=w357, "Wire Source"=w359) -> (reference out=w355:refnum<vi>, error out=w354:errorcluster)  [unwired: 4 in, 5 out]
                              n214 = property class="Term"(reference=w355, error in=w354) -> (error out=w351:errorcluster, "Wire"=w353:refnum<vi>)  [unwired: 1 out]
                              n215 = case shown="True" w349 {
                                tunnel: w356 -> [w376 _]
                                tunnel: w351 -> [_ _]
                                frame False {
                                n216 = Close Reference(reference=w376) -> ()  [unwired: 1 in, 1 out]
                                }
                                frame True {
                                }
                              }
                              n217 = invoke class="Wire" method="CleanUpWire"(reference=w353) -> (reference out=w352:refnum<vi>)  [unwired: 2 in, 2 out]
                              n218 = Close Reference(reference=w352) -> ()  [unwired: 1 in, 1 out]
                            }
                          }
                        }
                      }
                    }
                    n219 = stacked-sequence {
                      tunnel: w225 -> [w260]
                      tunnel: w221 -> [w259]
                      tunnel: [w255] -> w224
                      tunnel: w223 -> [w254]
                      frame #0 {
                        # "Remove the AlwaysCopyNode"
                        n220 = Index Array(array=w259) -> (element #1=w258:refnum<vi>, element #2=w257:refnum<vi>)  [unwired: 2 in]
                        n221 = invoke class="Term" method="Connect Wire"(reference=w258, error in=w260, "Wire Source"=w257) -> (error out=w256:errorcluster)  [unwired: 4 in, 6 out]
                        n222 = invoke class="Func" method="Delete"(reference=w254, error in=w256) -> (error out=w255:errorcluster)  [unwired: 1 in, 2 out]
                      }
                    }
                  }
                }
              }
              frame True {
              }
            }
            n223 = Close Reference(reference=w67) -> ()  [unwired: 1 in, 1 out]
            n224 = Close Reference(reference=w60) -> ()  [unwired: 1 in, 1 out]
            n225 = Close Reference(reference=w61) -> ()  [unwired: 1 in, 1 out]
            n226 = Close Reference(reference=w62) -> ()  [unwired: 1 in, 1 out]
            n227 = Close Reference(reference=w66) -> ()  [unwired: 1 in, 1 out]
            n228 = Close Reference(reference=w65) -> ()  [unwired: 1 in, 1 out]
            n229 = Close Reference(reference=w64) -> ()  [unwired: 1 in, 1 out]
          }
          frame False {
          }
        }
      }
      n230 = Close Reference(reference=w18) -> ()  [unwired: 1 in, 1 out]
      n231 = Close Reference(reference=w17) -> ()  [unwired: 1 in, 1 out]
      n232 = Close Reference(reference=w20) -> ()  [unwired: 1 in, 1 out]
    }
    frame Error {
    }
  }
  "error out" <- w4
  "ViRefOut" <- "ViRef"
